vi "fetchDataMN.vi"(8 "error in (no error)":errorcluster, 9 "node":string[](array[string]), 10 "shot":i32=1, 11 "treeName":string="emds") -> (0 "error out":errorcluster, 3 "data":dbl[][](array[numeric]))   [LabVIEW 2017]
uses:
  <vilib>/MDSplus/Library/MDSplus.lvlib
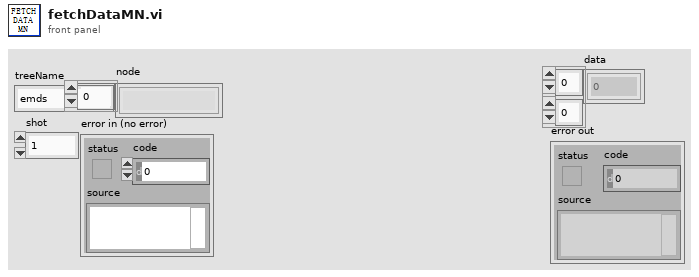
[diagram p1: front panel]
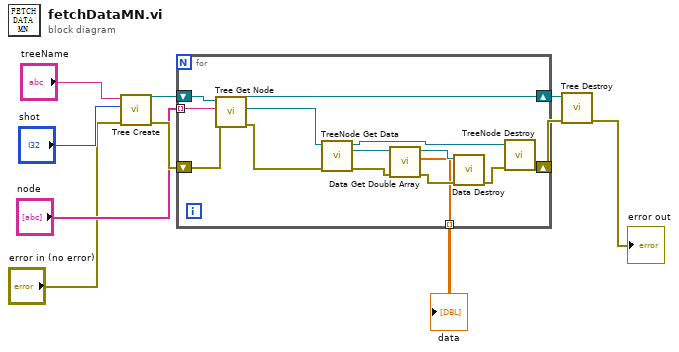
[diagram p0: block diagram]
diagram:
  n1 = call <vilib>:"Tree Create.vi"("error in (no error)"="error in (no error)", "Shot"="shot", "Name"="treeName") -> ("error out"=w9:errorcluster, "Tree DVR out"=w10:refnum<data-value>)  [unwired: 7 in]
  n2 = for {
    tunnel: "node" -> [w20] mode=indexing
    tunnel: [w11] -> w3 mode=indexing
    shift-right: [w22] -> w6
    shift-left: w10 -> [w24]
    shift-right: [w21] -> w5
    shift-left: w9 -> [w23]
    n3 = call <vilib>:"Tree Get Node.vi"("error in (no error)"=w23, "Path"=w20, "Tree DVR in"=w24) -> ("error out"=w18:errorcluster, "Node out"=w19:refnum<data-value>, "Tree DVR out"=w22:refnum<data-value>)  [unwired: 6 in]
    n4 = call <vilib>:"TreeNode Get Data.vi"("error in (no error)"=w18, "TreeNode DVR in"=w19) -> ("error out"=w12:errorcluster, "Data out"=w17:refnum<data-value>, "TreeNode DVR out"=w16:refnum<data-value>)  [unwired: 7 in]
    n5 = call <vilib>:"Data Get Double Array.vi"("error in (no error)"=w12, "Data DVR in"=w17) -> ("error out"=w14:errorcluster, "DBL array out"=w11:dbl[], "Data DVR out"=w15:refnum<data-value>)  [unwired: 6 in, 1 out]
    n6 = call <vilib>:"Data Destroy.vi"("error in (no error)"=w14, "Data DVR in"=w15) -> ("error out"=w13:errorcluster)  [unwired: 9 in]
    n7 = call <vilib>:"TreeNode Destroy.vi"("error in (no error)"=w13, "TreeNode DVR in"=w16) -> ("error out"=w21:errorcluster)  [unwired: 9 in]
  }
  "data" <- w3
  n8 = call <vilib>:"Tree Destroy.vi"("error in (no error)"=w5, "Tree DVR in"=w6) -> ("error out"=→"error out":errorcluster)  [unwired: 9 in]
